vi "Self Test.vi"(8 "error in":errorcluster, 11 "89XX in":refnum<class "89XX.lvclass">) -> (0 "error out":errorcluster, 3 "89XX out":refnum<class "89XX.lvclass">)   [LabVIEW 2019, in "89XX.lvlib" / "89XX.lvclass"]
doc: "This Override VI must be called by ancestor classes\nThis class reads error data and transmits it to the fault handler"
uses:
  Library/89XX.lvclass
  Library/89XX.lvclass/89XX.ctl
  builds/Instruments/PowerSupply.lvlibp/Library/PowerSupply.lvclass
  <instrlib>/Keysight N8900 Series/Keysight N8900 Series.lvlib
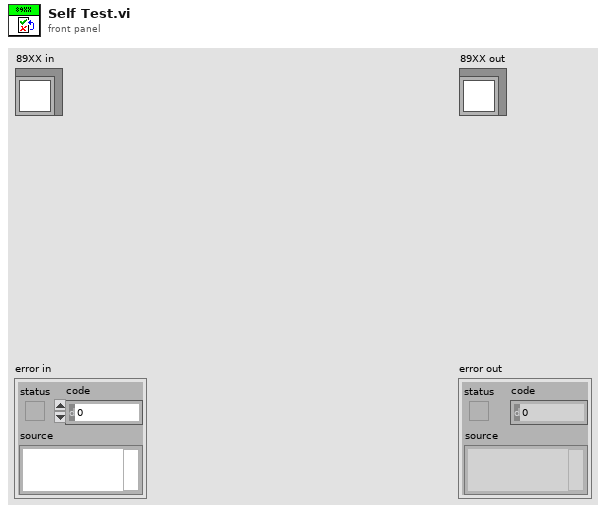
[diagram p1: front panel]
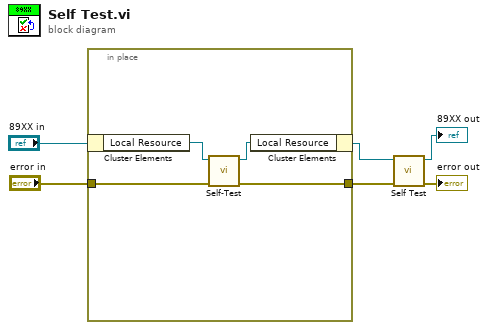
[diagram p0: block diagram]
diagram:
  n1 = in-place {
    in-place-border: "error in" -> [w8]
    in-place-border: [w7] -> w1
    n2 = in-place-cluster #1("89XX in") -> ("Local Resource"=w10:refnum<visa-resource-name>)
    n3 = call <instrlib>:"Self-Test.vi"("error in (no error)"=w8, "VISA resource name"=w10) -> ("error out"=w7:errorcluster, "VISA resource name out"=w9:refnum<visa-resource-name>)  [unwired: 6 in, 2 out]
    n4 = in-place-cluster #1("Local Resource"=w9) -> (w3:refnum<class "89XX.lvclass">)
  }
  n5 = call-parent "Self Test.vi"("error in"=w1, "Instruments in"=w3) -> ("error out"=→"error out":errorcluster, "Instruments out"=→"89XX out":refnum<class "89XX.lvclass">)  [unwired: 8 in]
